vi "BK Precision 983X Series Run List Program.vi"() -> ()   [LabVIEW 2015]
doc: "This example demonstrates how to setup and run a list program."
uses:
  <instrlib>/BK Precision 983X Series/BK Precision 983X Series.lvlib
panel:
  out "Actual DC Voltage Level (V)":dbl format="%.4g"
  out "Actual DC Current Level (A)":dbl format="%.4g"
  out "Output Frequency (Hz)":dbl format="%.4g"
  out "Actual AC Voltage Level (V)":dbl format="%.4g"
  out "Actual AC Current Level (A)":dbl format="%.4g"
  in  "stop":bool
  in  "Wave Variable (0)":u32 max=100
  in  "Waveform (0:Sine)":u16(ring) items=["Sine", "Square", "Clipped", "THD", "User"]
  in  "Select Output Waveform (0:Waveform A)":u16(ring) items=["Waveform A", "Waveform B"]
  in  "List Location (0)":u32 max=9 format="%#_0f"
  in  "VISA resource name":refnum<visa-resource-name>
  # "(c) 2017 B&K Precision Corporation.  ALL RIGHTS RESERVED."
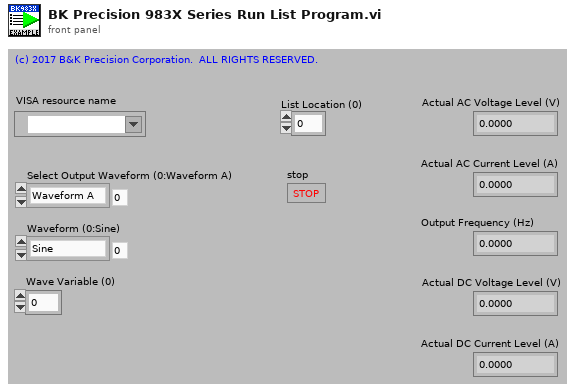
[diagram p1: front panel]
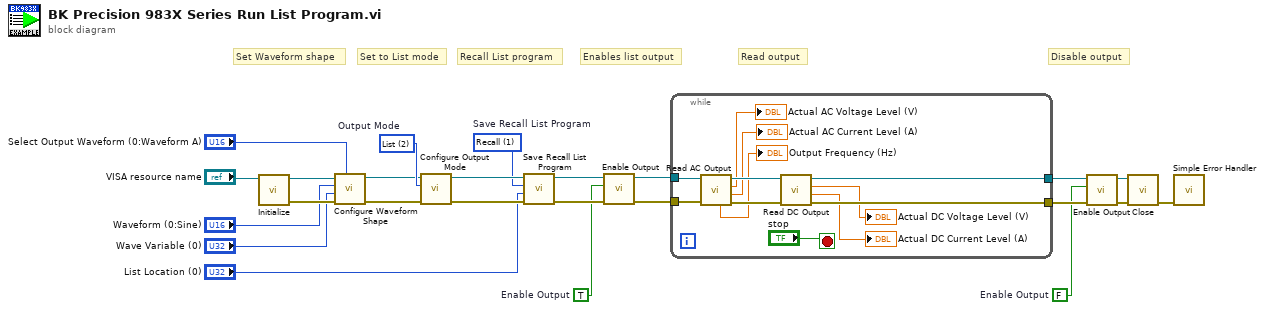
[diagram p0: block diagram]
diagram:
  w1 = FALSE  # Enable Output
  w8 = TRUE  # Enable Output
  w19 = u16 1 items=["Save", "Recall"]  # Save Recall List Program
  w22 = u16 2 items=["Normal", "Step", "List", "Pulse"]  # Output Mode
  # "Disable output"
  # "Read output"
  # "Set Waveform shape"
  # "Recall List program"
  # "Set to List mode"
  # "Enables list output"
  n1 = call <instrlib>:"Initialize.vi"("VISA resource name"="VISA resource name") -> ("error out"=w13:errorcluster, "VISA resource name out"=w14:refnum<visa-resource-name>)  [unwired: 9 in]
  n2 = call <instrlib>:"Configure Waveform Shape.vi"("Select Output Waveform (0:Waveform A)"="Select Output Waveform (0:Waveform A)", "error in (no error)"=w13, "Wave Variable (0)"="Wave Variable (0)", "Waveform (0:Sine)"="Waveform (0:Sine)", "VISA resource name"=w14) -> ("error out"=w15:errorcluster, "VISA resource name out"=w16:refnum<visa-resource-name>)  [unwired: 5 in]
  n3 = call <instrlib>:"Configure Output Mode.vi"("error in (no error)"=w15, "Output Mode (0:Normal)"=w22, "VISA resource name"=w16) -> ("error out"=w20:errorcluster, "VISA resource name out"=w21:refnum<visa-resource-name>)  [unwired: 7 in]
  n4 = call <instrlib>:"Save Recall List Program.vi"("error in (no error)"=w20, "List Location (0)"="List Location (0)", "Save Recall List Program (0:Save)"=w19, "VISA resource name"=w21) -> ("error out"=w9:errorcluster, "VISA resource name out"=w10:refnum<visa-resource-name>)  [unwired: 6 in]
  n5 = call <instrlib>:"Enable Output.vi"("error in (no error)"=w9, "Enable Output (F: False)"=w8, "VISA resource name"=w10) -> ("error out"=w6:errorcluster, "VISA resource name out"=w7:refnum<visa-resource-name>)  [unwired: 7 in]
  n6 = while {
    tunnel: w7 -> [w35]
    tunnel: w6 -> [w34]
    tunnel: [w31] -> w3
    tunnel: [w30] -> w2
    stop <- "stop" stop-if-true
    n7 = call <instrlib>:"Read AC Output.vi"("error in (no error)"=w34, "VISA resource name"=w35) -> ("error out"=w32:errorcluster, "Actual AC Current Level (A)"=→"Actual AC Current Level (A)":dbl, "Actual AC Voltage Level (V)"=→"Actual AC Voltage Level (V)":dbl, "VISA resource name out"=w33:refnum<visa-resource-name>, "Output Frequency (Hz)"=→"Output Frequency (Hz)":dbl)  [unwired: 5 in]
    n8 = call <instrlib>:"Read DC Output.vi"("error in (no error)"=w32, "VISA resource name"=w33) -> ("error out"=w30:errorcluster, "Actual DC Current Level (A)"=→"Actual DC Current Level (A)":dbl, "Actual DC Voltage Level (V)"=→"Actual DC Voltage Level (V)":dbl, "VISA resource name out"=w31:refnum<visa-resource-name>)  [unwired: 6 in]
  }
  n9 = call <instrlib>:"Enable Output.vi"("error in (no error)"=w2, "Enable Output (F: False)"=w1, "VISA resource name"=w3) -> ("error out"=w4:errorcluster, "VISA resource name out"=w5:refnum<visa-resource-name>)  [unwired: 7 in]
  n10 = call <instrlib>:"Close.vi"("error in (no error)"=w4, "VISA resource name"=w5) -> ("error out"=w23:errorcluster)  [unwired: 9 in]
  n11 = call <vilib>:"Simple Error Handler.vi"("error in (no error)"=w23) -> ()  [unwired: 4 in, 5 out]
